vi "Frame Page.vi"(8 "error in (no error)":errorcluster, 11 "Node Ptr":T2 format="%.0x") -> (0 "error out":errorcluster)   [LabVIEW 2023, in "J1939 Addon System Explorer.lvlib"]
uses:
  J1939 Addon System Explorer.lvlib
  <vilib>/NI VeriStand/Custom Device API/Custom Device Item Ref.ctl
  NationalInstruments.VeriStand.SystemStorageUI
  Addon Shared/Types/Outgoing Event Trigger Types.ctl
  <vilib>/NI VeriStand/UI Controls/Single Node Browser/Net Event Data.ctl
  <vilib>/NI VeriStand/UI Controls/Single Node Browser/Net Event.ctl
  Support Libraries/J1939 Utilities/SubVIs/Convert CAN Arb ID to J1939 ID.vi
  Addon Shared/SubVIs/Constants.vi
  <vilib>/NI VeriStand/Custom Device API/Custom Device API.lvlib
  Support Libraries/J1939 Utilities/J1939 Utilities.lvlib
  Addon Shared/J1939 Addon Shared.lvlib
  <vilib>/NI VeriStand/UI Controls/Single Node Browser/NI_VS UI Single Node Browser.lvlib
panel:
  in  "Transmit Trigger":T1
  in  "Trigger":refnum<k24>(container)
  in  "Trigger Settings":cluster{"Section Name":string}={"Section Name"="Transmission Trigger"}
  in  "Trigger":refnum<k24>(container)
  in  "Disable Transmission":bool
  in  "Disable Settings":cluster{"Section Name":string}={"Section Name"="Disable Transmission"}
  in  "Description":string
  out "Source Address":u8 format="%.0x"
  out "Priority":u8 format="%.0x"
  out "PGN":u32 format="%.0x"
  out "Frame ID":u32 format="%.0x"
  in  "Custom Device Settings":cluster{"Section Name":string}={"Section Name"="Frame Settings"}
  out "Name":string
  in  "SHDocVw.IWebBrowser2":refnum<k7>(container)
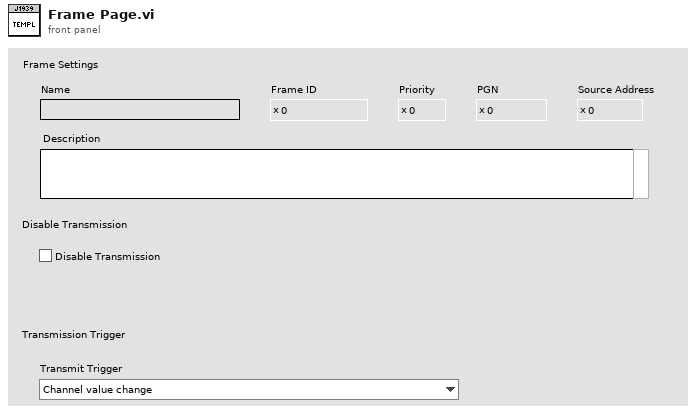
[diagram p1: front panel]
types:
  T1 = typedef "J1939 Addon Shared.lvlib/Outgoing Event Trigger Types.ctl" = enum16{"Channel value change", "Trigger channel (not zero)", "Channel value change or trigger channel (not zero)", "Trigger channel (any value change)", "Channel value change or trigger channel (any value change)"}
  T2 = typedef "Custom Device API.lvlib/Custom Device Item Ref.ctl" = u64
  T3 = cluster{"Trigger":refnum<user-event>, "Transmission":refnum<user-event>}
  T4 = typedef "J1939 Addon Shared.lvlib/Frame.Settings.ctl" = cluster{"ID":u32, "Disable Transmission":bool, "Disable Transmission Ref":T2, "Transmit Trigger":T1, "Transmit Trigger Ref":T2}
  T5 = typedef "Custom Device API.lvlib/Custom Device Item Info.ctl" = cluster{"Name":string, "Is Channel":bool, "GUID":string, "Is Waveform":bool}
  T6 = typedef "NI_VS UI Single Node Browser.lvlib/Single Node Browser Ref.ctl" = refnum<k24>
  T7 = typedef "NI_VS UI Single Node Browser.lvlib/Callback Type.ctl" = cluster{"Net Callbacks":refnum<k27>[], "Event":refnum<user-event>}
  T8 = typedef "Custom Device API.lvlib/Custom Device Commands.ctl" = enum16{"Default", "Item renamed", "Shutdown", "Dynamic button pressed"}
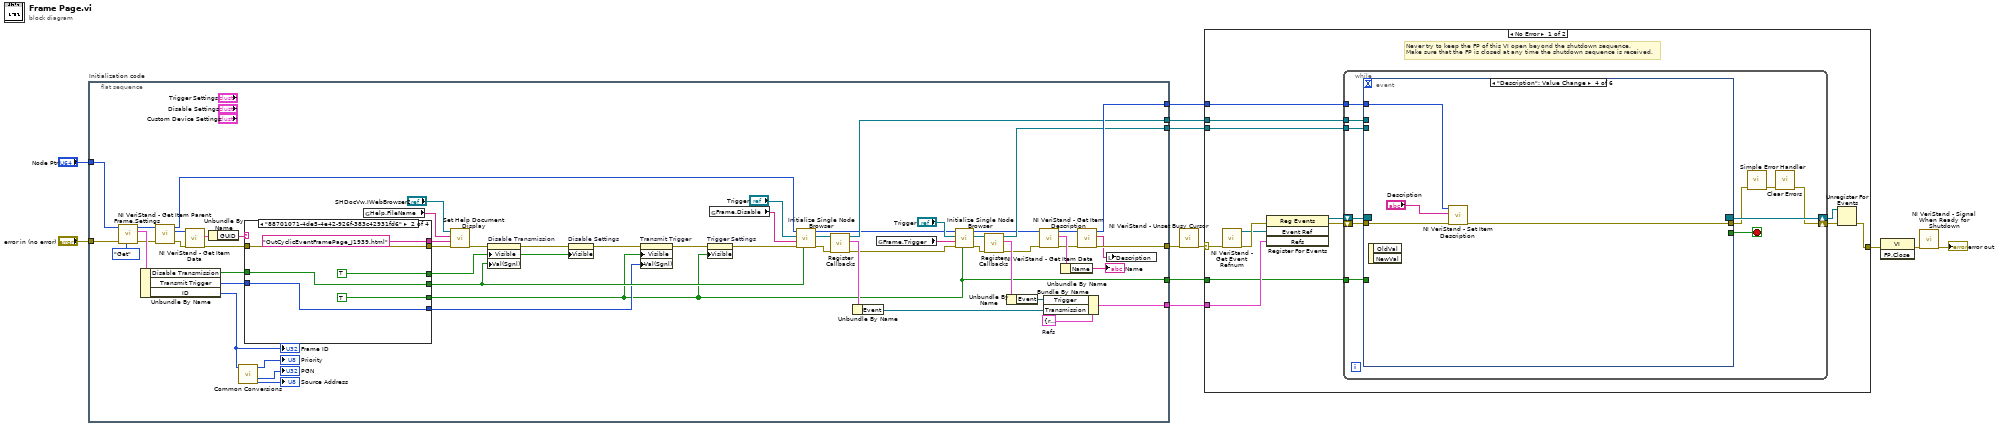
[diagram p0: block diagram]
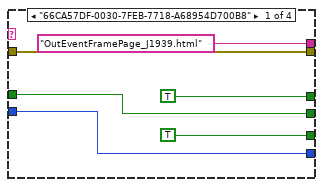
[diagram p2: hidden frame]
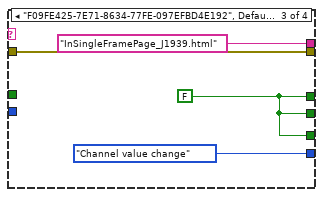
[diagram p3: hidden frame]
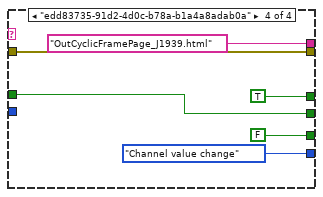
[diagram p4: hidden frame]
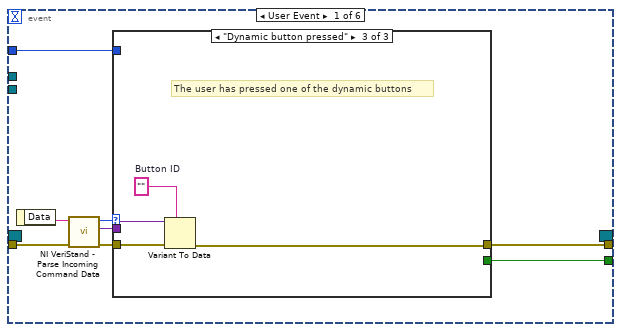
[diagram p5: hidden frame]
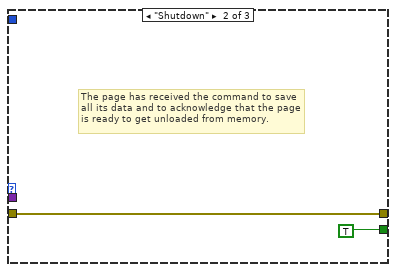
[diagram p7: hidden frame]
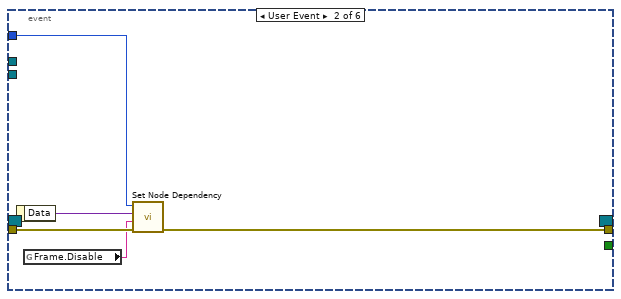
[diagram p8: hidden frame]
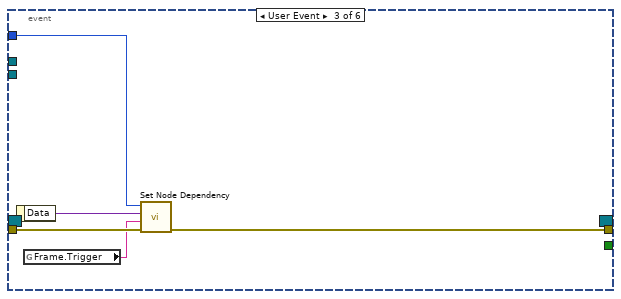
[diagram p9: hidden frame]
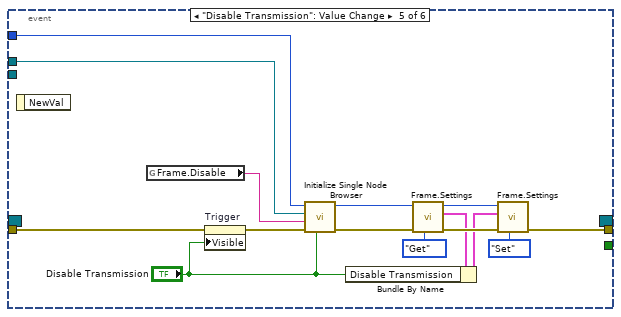
[diagram p10: hidden frame]
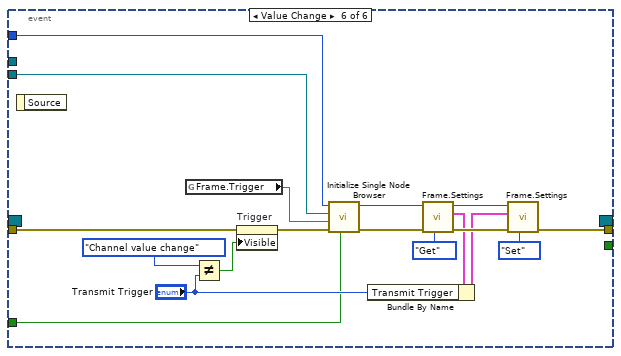
[diagram p11: hidden frame]
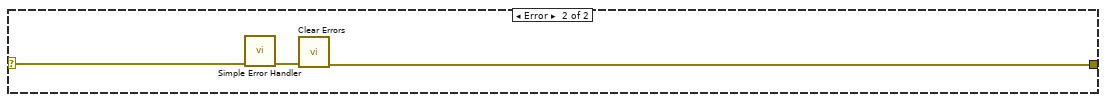
[diagram p12: hidden frame]
diagram:
  n1 = flat-sequence "Initialization code" {
    tunnel: "error in (no error)" -> [w21]
    tunnel: "Node Ptr" -> [w19]
    tunnel: [w62] -> w7
    tunnel: [w60] -> w5
    tunnel: [w43] -> w4
    tunnel: [w46] -> w3
    tunnel: [w34] -> w2
    tunnel: [w14] -> w1
    frame #0 {
      w38 = T3 {"Trigger"=refnum, "Transmission"=refnum}  # Refs
      n2 = call "Frame.Settings.vi"("Action"=enum8{"Get", "Set"}."Get", "error in (no error)"=w21, "Item Ref in"=w19) -> ("error out"=w20:errorcluster, "Frame.Settings"=w25:T4, "Item Ref out"=w18:T2)  [unwired: 6 in]
      n3 = Unbundle By Name(w25) -> ("Disable Transmission"=w17:bool, "Transmit Trigger"=w16:T1, "ID"=w24:u32)
      "Frame ID" <- w24
      n4 = call <vilib>:"NI VeriStand - Get Item Parent.vi"("error in (no error)"=w20, "Item Ref in"=w18) -> ("error out"=w58:errorcluster, "Parent Ref"=w57:T2, "Item Ref out"=w50:T2)  [unwired: 6 in, 1 out]
      n5 = call <vilib>:"NI VeriStand - Get Item Data.vi"("error in (no error)"=w58, "Item Ref in"=w57) -> ("error out"=w54:errorcluster, "Item Info"=w56:T5)  [unwired: 8 out]
      n6 = Unbundle By Name(w56) -> ("GUID"=w55:string)
      n7 = call-poly "Common Conversions.vi"("Arb ID"=w24) -> ("Priority"=→"Priority":u8, "PGN"=→"PGN":u32, "Source Address"=→"Source Address":u8)  [unwired: 11 in, 1 out]
      n8 = case shown="\"88701071-4de5-4e42-926f-383c42931fd6\"" w55 {
        tunnel: ["OutEventFramePage_J1939.html" ("HTML File") "OutCyclicEventFramePage_J1939.html" ("HTML File") "InSingleFramePage_J1939.html" ("HTML File") "OutCyclicFramePage_J1939.html" ("HTML File")] -> w69
        tunnel: w54 -> [w75 w81 w85 w91]
        tunnel: [w75 w81 w85 w91] -> w27
        tunnel: [TRUE TRUE w84 TRUE] -> w47
        tunnel: [w71 w77 w84 w88] -> w29
        tunnel: [TRUE TRUE w84 FALSE] -> w14
        tunnel: [w72 w78 Outgoing_Event_Trigger_Types."Channel value change" ("y") Outgoing_Event_Trigger_Types."Channel value change" ("y")] -> w28
        tunnel: w17 -> [w71 w77 _ w88]
        tunnel: w16 -> [w72 w78 _ _]
        frame "66CA57DF-0030-7FEB-7718-A68954D700B8" {
        }
        frame "88701071-4de5-4e42-926f-383c42931fd6" {
        }
        frame "F09FE425-7E71-8634-77FE-097EFBD4E192", Default {
          w84 = FALSE
        }
        frame "edd83735-91d2-4d0c-b78a-b1a4a8adab0a" {
        }
      }
      n9 = global read "Constants.vi" "Help.FileName"() -> (w13:string)
      n10 = call "Set Help Document Display.vi"("error in (no error)"=w27, "HTML File"=w69, "Main CHM File"=w13, "SHDocVw.IWebBrowser2"="SHDocVw.IWebBrowser2") -> ("error out"=w26:errorcluster)  [unwired: 7 in]
      n11 = property on="Disable Transmission" class="Bool (strict)"(error in=w26, "Visible"=w47, "Val(Sgnl)"=w29) -> (error out=w53:errorcluster)  [unwired: 1 in, 1 out]
      n12 = property on="Disable Settings" class="Clust (strict)"(error in=w53, "Visible"=w47) -> (error out=w31:errorcluster)  [unwired: 1 in, 1 out]
      n13 = property on="Transmit Trigger" class="Enum (strict)"(error in=w31, "Visible"=w14, "Val(Sgnl)"=w28) -> (error out=w30:errorcluster)  [unwired: 1 in, 1 out]
      n14 = property on="Trigger Settings" class="Clust (strict)"(error in=w30, "Visible"=w14) -> (error out=w32:errorcluster)  [unwired: 1 in, 1 out]
      n15 = global read "Constants.vi" "Frame.Disable"() -> (w45:string)
      n16 = call "Initialize Single Node Browser.vi"("Use Channel?"=w29, "error in (no error)"=w32, "NodeName"=w45, "Browser Ref 2"="Trigger", "Item Ref in"=w50) -> ("error out"=w52:errorcluster, "Browser Ref"=w51:T6, "Item Ref out"=w33:T2)  [unwired: 4 in]
      n17 = call <vilib>:"Register Callbacks.vi"("error in (no error)"=w52, "Single Node Browser"=w51) -> ("error out"=w39:errorcluster, "Callbacks"=w49:T7, "Single Node Browser dup"=w46:T6)  [unwired: 7 in]
      n18 = Unbundle By Name(w49) -> ("Event"=w44:refnum<user-event>)
      n19 = global read "Constants.vi" "Frame.Trigger"() -> (w36:string)
      n20 = call "Initialize Single Node Browser.vi"("Use Channel?"=w14, "error in (no error)"=w39, "NodeName"=w36, "Browser Ref 2"="Trigger", "Item Ref in"=w33) -> ("error out"=w40:errorcluster, "Browser Ref"=w41:T6, "Item Ref out"=w22:T2)  [unwired: 4 in]
      n21 = call <vilib>:"Register Callbacks.vi"("error in (no error)"=w40, "Single Node Browser"=w41) -> ("error out"=w23:errorcluster, "Callbacks"=w42:T7, "Single Node Browser dup"=w34:T6)  [unwired: 7 in]
      n22 = Unbundle By Name(w42) -> ("Event"=w37:refnum<user-event>)
      n23 = call <vilib>:"NI VeriStand - Get Item Data.vi"("error in (no error)"=w23, "Item Ref in"=w22) -> ("error out"=w63:errorcluster, "Item Info"=w68:T5, "Item Ref out"=w61:T2)  [unwired: 7 out]
      n24 = Bundle By Name(cluster=w38, "Trigger"=w37, "Transmission"=w44) -> (w43:T3)
      n25 = Unbundle By Name(w68) -> ("Name"=→"Name":string)
      n26 = call <vilib>:"NI VeriStand - Get Item Description.vi"("error in (no error)"=w63, "Item Ref in"=w61) -> ("error out"=w62:errorcluster, "Description"=w59:string, "Item Ref out"=w60:T2)  [unwired: 7 out]
      n27 = local write "Description"(w59) -> ()
    }
  }
  n28 = call <vilib>:"NI VeriStand - Unset Busy Cursor.vi"("error in (no error)"=w7) -> ("error out"=w9:errorcluster)  [unwired: 10 out]
  n29 = case shown="No Error" w9 {
    selector: w9 -> [w97 w181]
    tunnel: [w102 w179] -> w12
    tunnel: w5 -> [w98 _]
    tunnel: w4 -> [w96 _]
    tunnel: w3 -> [w95 _]
    tunnel: w2 -> [w94 _]
    tunnel: w1 -> [w93 _]
    frame No Error {
      # "Never try to keep the FP of this VI open beyond the shutdown sequence.\nMake sure that the FP is closed at any time the shutdown sequence is received."
      n30 = call <vilib>:"NI VeriStand - Get Event Refnum.vi"("error in (no error)"=w97) -> ("error out"=w105:errorcluster, "Event Ref"=w101:refnum<user-event>)  [unwired: 9 out]
      n31 = register-events(error in=w105, w101, w96) -> (reference out=w99:refnum<event-registration>, error out=w100:errorcluster)  [unwired: 1 in]
      n32 = while {
        tunnel: w98 -> [w112]
        shift-right: [w109] -> w103
        shift-left: w100 -> [w115]
        shift-right: [w116] -> w104
        shift-left: w99 -> [w114]
        tunnel: w95 -> [w108]
        tunnel: w94 -> [w107]
        tunnel: w93 -> [w106]
        stop <- w113 stop-if-true
        n33 = event shown="[3] \"Description\": Value Change" {
          selector: w114 -> [_ _ _ _ _ _]
          dyn-events: [_ _ _ _ _ _] -> w116
          timeout: _ -> [_ _ _ _ _ _]
          tunnel: w115 -> [w124 w134 w139 w145 w160 w178]
          tunnel: [w120 _ _ _ _ _] -> w113
          tunnel: [w119 w133 w138 w144 w150 w164] -> w111
          tunnel: w112 -> [w118 w135 w140 w143 w158 w177]
          tunnel: w108 -> [_ _ _ _ w159 _]
          tunnel: w107 -> [_ _ _ _ _ w172]
          tunnel: w106 -> [_ _ _ _ _ w162]
          event User Event {
            n34 = event-data() -> ("Data"=w123:string)  [unwired: 1 out]
            n35 = call <vilib>:"NI VeriStand - Parse Incoming Command Data.vi"("error in (no error)"=w124, "Incoming data"=w123) -> ("error out"=w122:errorcluster, "Outgoing data"=w117:variant, "Action"=w121:T8)  [unwired: 7 out]
            n36 = case shown="\"Dynamic button pressed\"" w121 {
              tunnel: w122 -> [w125 w126 w131]
              tunnel: [_ TRUE _] -> w120
              tunnel: [w125 w126 w128] -> w119
              tunnel: w118 -> [_ _ _]
              tunnel: w117 -> [_ _ w130]
              frame "Default", Default {
              }
              frame "Shutdown" {
                # "The page has received the command to save all its data and to acknowledge that the page is ready to get unloaded from memory."
              }
              frame "Dynamic button pressed" {
                w129 = ""  # Button ID
                # "The user has pressed one of the dynamic buttons"
                n37 = Variant To Data(error in=w131, type=w129, Variant=w130) -> (error out=w128:errorcluster)  [unwired: 1 out]
              }
            }
          }
          event User Event {
            n38 = event-data() -> ("Data"=w136:variant)  [unwired: 1 out]
            n39 = global read "Constants.vi" "Frame.Disable"() -> (w132:string)
            n40 = call "Set Node Dependency.vi"("error in (no error)"=w134, "NodeName"=w132, "Data"=w136, "Item Ref in"=w135) -> ("error out"=w133:errorcluster)  [unwired: 6 in, 1 out]
          }
          event User Event {
            n41 = event-data() -> ("Data"=w141:variant)  [unwired: 1 out]
            n42 = global read "Constants.vi" "Frame.Trigger"() -> (w137:string)
            n43 = call "Set Node Dependency.vi"("error in (no error)"=w139, "NodeName"=w137, "Data"=w141, "Item Ref in"=w140) -> ("error out"=w138:errorcluster)  [unwired: 6 in, 1 out]
          }
          event "Description": Value Change {
            n44 = event-data() -> ()  [unwired: 3 out]
            n45 = call <vilib>:"NI VeriStand - Set Item Description.vi"("error in (no error)"=w145, "Description"="Description", "Item Ref in"=w143) -> ("error out"=w144:errorcluster)  [unwired: 8 out]
          }
          event "Disable Transmission": Value Change {
            n46 = event-data() -> ()  [unwired: 2 out]
            n47 = global read "Constants.vi" "Frame.Disable"() -> (w156:string)
            n48 = property on="Trigger" class="AXCont"(error in=w160, "Visible"="Disable Transmission") -> (error out=w157:errorcluster)  [unwired: 1 in, 1 out]
            n49 = call "Initialize Single Node Browser.vi"("Use Channel?"="Disable Transmission", "error in (no error)"=w157, "NodeName"=w156, "Browser Ref 2"=w159, "Item Ref in"=w158) -> ("error out"=w153:errorcluster, "Item Ref out"=w154:T2)  [unwired: 4 in, 1 out]
            n50 = call "Frame.Settings.vi"("Action"=enum8{"Get", "Set"}."Get", "error in (no error)"=w153, "Item Ref in"=w154) -> ("error out"=w151:errorcluster, "Frame.Settings"=w148:T4, "Item Ref out"=w149:T2)  [unwired: 6 in]
            n51 = Bundle By Name(cluster=w148, "Disable Transmission"="Disable Transmission") -> (w146:T4)
            n52 = call "Frame.Settings.vi"("Action"=enum8{"Get", "Set"}."Set", "error in (no error)"=w151, "Frame.Settings"=w146, "Item Ref in"=w149) -> ("error out"=w150:errorcluster)  [unwired: 5 in, 2 out]
          }
          event Value Change {
            n53 = event-data() -> ()  [unwired: 2 out]
            n54 = global read "Constants.vi" "Frame.Trigger"() -> (w175:string)
            n55 = Not Equal?(x=Outgoing_Event_Trigger_Types."Channel value change" ("y"), y="Transmit Trigger") -> (x != y?=w173:bool)
            n56 = property on="Trigger" class="AXCont"(error in=w178, "Visible"=w173) -> (error out=w176:errorcluster)  [unwired: 1 in, 1 out]
            n57 = call "Initialize Single Node Browser.vi"("Use Channel?"=w162, "error in (no error)"=w176, "NodeName"=w175, "Browser Ref 2"=w172, "Item Ref in"=w177) -> ("error out"=w165:errorcluster, "Item Ref out"=w163:T2)  [unwired: 4 in, 1 out]
            n58 = call "Frame.Settings.vi"("Action"=enum8{"Get", "Set"}."Get", "error in (no error)"=w165, "Item Ref in"=w163) -> ("error out"=w169:errorcluster, "Frame.Settings"=w167:T4, "Item Ref out"=w168:T2)  [unwired: 6 in]
            n59 = Bundle By Name(cluster=w167, "Transmit Trigger"="Transmit Trigger") -> (w161:T4)
            n60 = call "Frame.Settings.vi"("Action"=enum8{"Get", "Set"}."Set", "error in (no error)"=w169, "Frame.Settings"=w161, "Item Ref in"=w168) -> ("error out"=w164:errorcluster)  [unwired: 5 in, 2 out]
          }
        }
        n61 = call <vilib>:"Simple Error Handler.vi"("error in (no error)"=w111) -> ("error out"=w110:errorcluster)  [unwired: 1 in, 7 out]
        n62 = call <vilib>:"Clear Errors.vi"("error in (no error)"=w110) -> ("error out"=w109:errorcluster)  [unwired: 1 in, 5 out]
      }
      n63 = Unregister For Events(event registration refnum=w104, error in=w103) -> (error out=w102:errorcluster)
    }
    frame Error {
      n64 = call <vilib>:"Simple Error Handler.vi"("error in (no error)"=w181) -> ("error out"=w180:errorcluster)  [unwired: 1 in, 7 out]
      n65 = call <vilib>:"Clear Errors.vi"("error in (no error)"=w180) -> ("error out"=w179:errorcluster)  [unwired: 1 in, 5 out]
    }
  }
  n66 = invoke class="VI" method="FP.Close"(error in=w12) -> (error out=w11:errorcluster)  [unwired: 2 in, 2 out]
  n67 = call <vilib>:"NI VeriStand - Signal When Ready for Shutdown.vi"("error in (no error)"=w11) -> ("error out"=→"error out":errorcluster)  [unwired: 10 out]
